vi "SigGenPwrMtr2.vi"() -> ()   [LabVIEW 2009]
uses:
  Reversing_Switch.ctl
panel:
  out "Noise Source Verified":bool
  in  "Inside Noise Source":bool
  in  "mSec":i32=250
  out "Power returned (dBm)":dbl(graph)=-33.1308036
  in  "stop":bool
  in  "Tab Control":T1(tab)=enum."SWITCH SETTINGS"
  out "RF Power":bool
  in  "RF ON/OFF":bool
  in  "Power Level (dB)":dbl=-120.0
  in  "Frequency (GHz)":dbl=2.809
  in  "SigGen Settings":bool
  out "Freq (GHz)":dbl=2809000000.0 format="%#_10e"
  out "Power":dbl=-120.0
  out "SigGen Errors":errorcluster
  in  "Switch Settings":bool
  in  "IO Switch #2 Output":T2(ring)
  in  "Signal Out Input":T3(ring)
  in  "Signal Out Output":T4(ring)
  in  "Power Meter Switch Input":T5(ring)
  in  "Amplifier Switch":enum16{"Bypass Amp", "Include Amp"}(ring)
  out "Reversing Switch":bool=TRUE
  out "IO Switch #1":bool=TRUE
  out "IO Switch #2":bool=TRUE
  out "Signal Out":bool=TRUE
  out "Signal Source":bool=TRUE
  out "Power Meter":bool=TRUE
  out "Amp By Pass":bool=TRUE
  in  "Reversing Switch":T6
  in  "IO Swith #2 Input":T7(ring)
  in  "IO Switch #1 Input":T8(ring)
  in  "Power Meter Switch Output":T9(ring)
  in  "Signnal Source Input":T10(ring)
  in  "Signal Source Output":T11(ring)
  in  "IO Switch #1 Output":T12(ring)
  out "Switch Errors":errorcluster
  in  "Attenuator Settings":bool
  in  "121 dB Attenuator":i32=121 min=0 max=121 step=1
  out "Active 121 dB Attenuators":bool[](array[boolean])=[FALSE, TRUE, TRUE, TRUE, TRUE, TRUE, TRUE, TRUE, TRUE]
  in  "70 dB Attenuator":i32=70 min=0 max=70 step=10
  out "Active 70 dB Attenuators":bool[](array[boolean])=[FALSE, TRUE, TRUE, TRUE]
  out "Attenuator Errors":errorcluster
  # "1 dB"
  # "2 dB"
  # "4 dB"
  # "4 dB"
  # "10 dB"
  # "20 dB"
  # "40 dB"
  # "40 dB"
  # "10 dB"
  # "20 dB"
  # "40 dB"
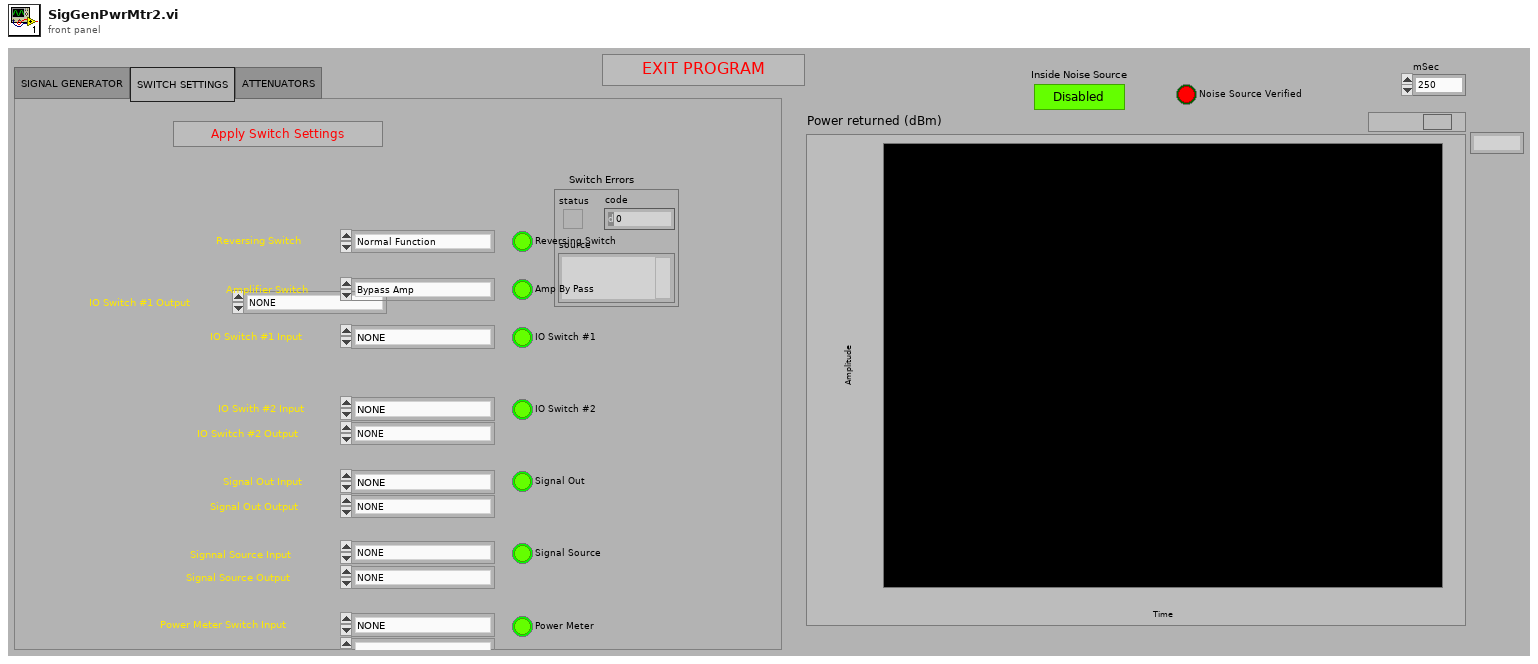
[diagram p1: front panel]
types:
  T1 = enum32{"SIGNAL GENERATOR", "SWITCH SETTINGS", "ATTENUATORS"}
  T2 = enum16{"NONE", "AVR (J3)", "Signal Out Switch (S3)", "Power Meter Switch (S5)", "Reversing Switch", "2W Term (TM1)"}
  T3 = enum16{"NONE", "Amp Bypass Switch (S6)", "IO Switch #1 (S1)", "IO Switch #2 (S2)", "2W Term (TM3)"}
  T4 = enum16{"NONE", "2 Watt Term (TM3)", "Splitter", "Power Meter Switch (S5)"}
  T5 = enum16{"NONE", "IO Switch #1 (S1)", "Signal Source Switch (S4)", "Signal Out Switch (S3)", "IO Switch #2 (S2)", "TXH-TXV Switch (J8)"}
  T6 = typedef "Reversing_Switch.ctl" = enum16{"Normal Function", "Reversing Function"}
  T7 = enum16{"NONE", "AVR (J3)", "Splitter", "Signal Out Switch (S3)", " 2W Term (TM1)", "Reversing Switch", "Power Meter Switch"}
  T8 = enum16{"NONE", "AHR (J2)", "Splitter", "Signal Out Switch (S3)", "Reversing Switch", "Power Meter Switch"}
  T9 = enum16{"NONE", "Power Meter (J6)", "IO Switch # 1", "IO Switch # 2"}
  T10 = enum16{"NONE", "Delay Device", "Signal Generator (J7)", "Inside Noise Box NF (J5)", "2W Term (TM3)"}
  T11 = enum16{"NONE", "Amp Bypass Switch", "Test Pulse Generator", "Power Meter Switch (S5)"}
  T12 = enum16{"NONE", "AHR (J2)", "Delay Device (S4)", "Power Meter Switch (S5)", "Reversing Switch"}
  T13 = enum16{"N1911A", "Siggen", "34980a", "E4418B", "Rvp8"}
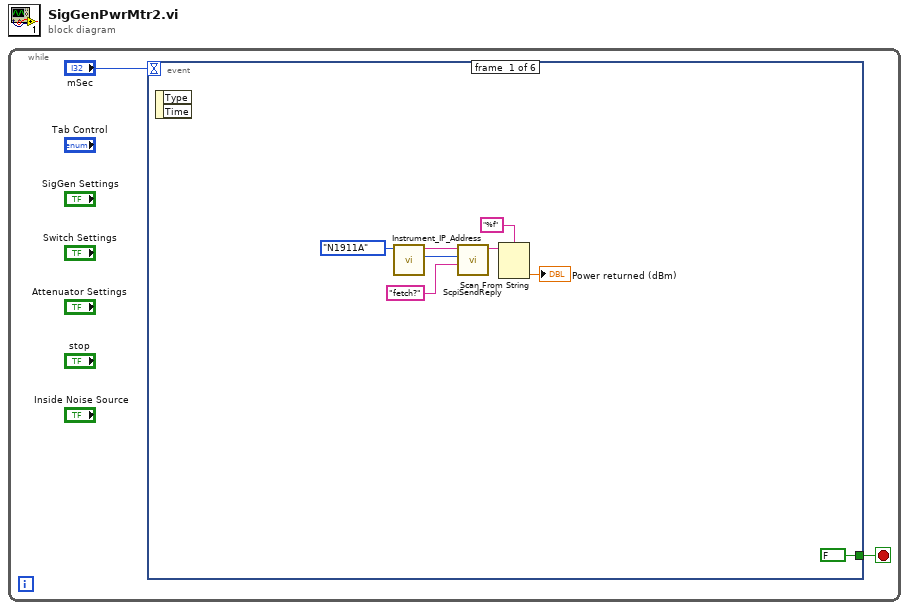
[diagram p0: block diagram]
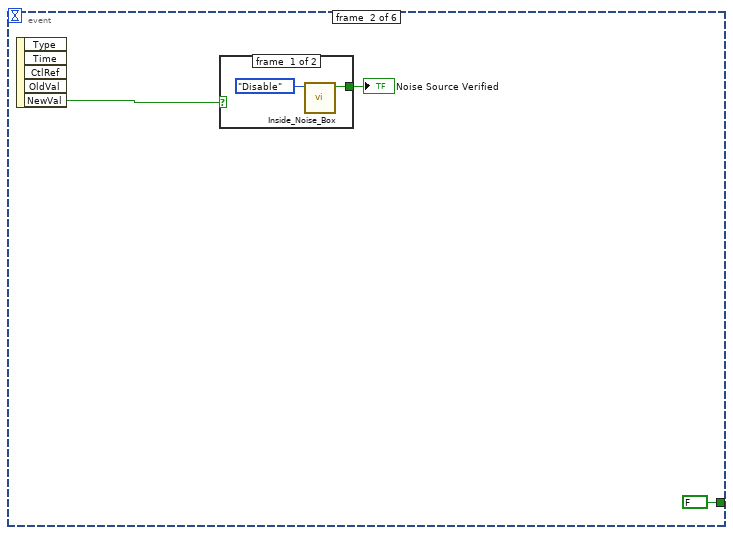
[diagram p2: hidden frame]
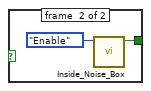
[diagram p3: hidden frame]
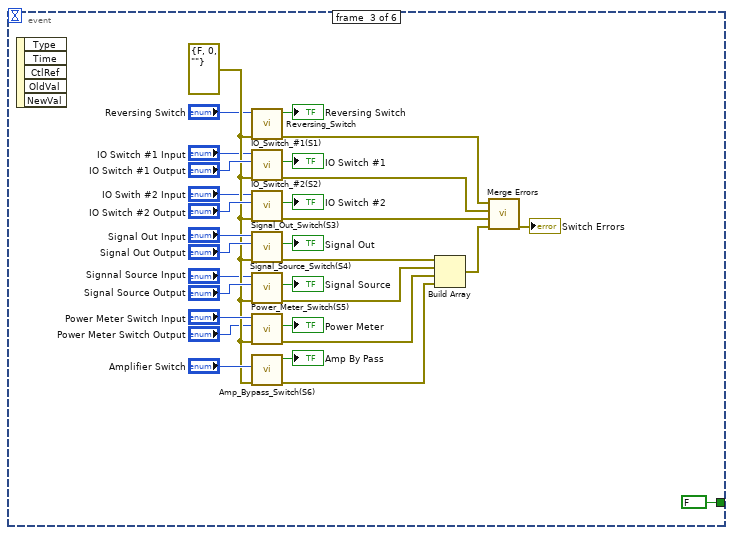
[diagram p4: hidden frame]
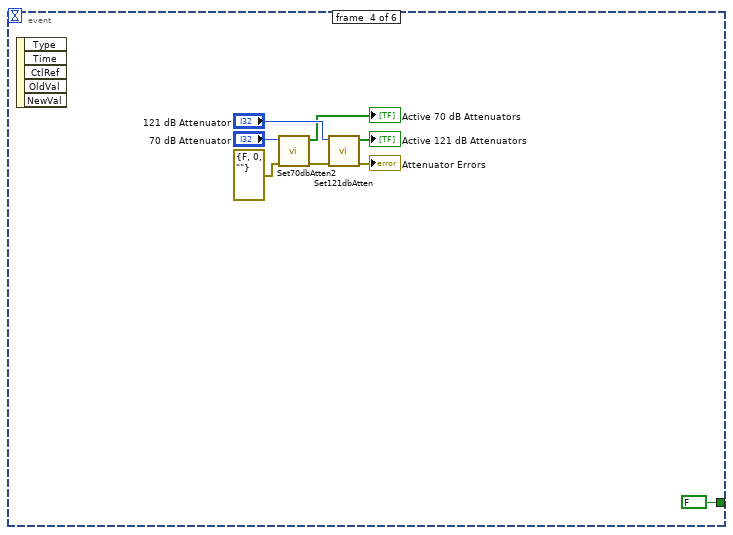
[diagram p5: hidden frame]
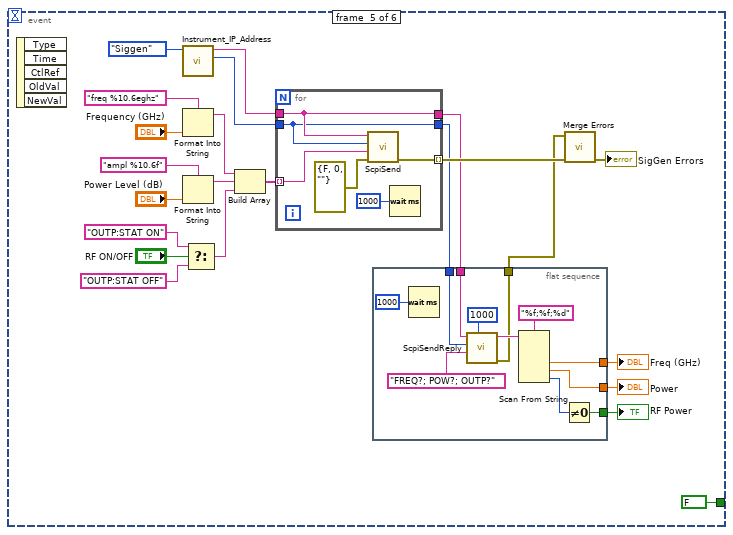
[diagram p6: hidden frame]
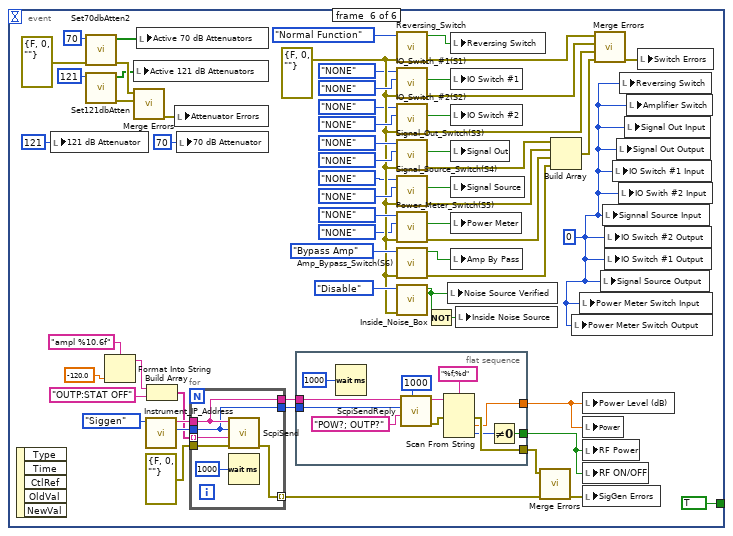
[diagram p7: hidden frame]
diagram:
  n1 = while {
    stop <- w2 stop-if-true
    n2 = event shown="[5] \"stop\": Value Change" {
      selector: _ -> [_ _ _ _ _ _]
      dyn-events: _ -> [_ _ _ _ _ _]
      timeout: "mSec" -> [_ _ _ _ _ _]
      tunnel: [FALSE FALSE FALSE FALSE FALSE TRUE] -> w2
      event #0 {
        n3 = event-data() -> ()  [unwired: 1 in, 2 out]
        n4 = call "Instrument_IP_Address.vi"("Instrument"=T13."N1911A") -> ("Port"=w10:u16, "IP Address"=w9:string)  [unwired: 9 in]
        n5 = call "ScpiSendReply.vi"("Command"="fetch?" ("format string"), "TCP port"=w10, "IP Address"=w9) -> ("Reply"=w5:string)  [unwired: 6 in, 1 out]
        n6 = Scan From String(format string="%f", input string=w5) -> (output 1=→"Power returned (dBm)":dbl)  [unwired: 3 in, 3 out]
      }
      event #1 {
        n7 = event-data() -> ("NewVal"=w13:bool)  [unwired: 1 in, 4 out]
        n8 = case shown="False" w13 {
          tunnel: [w14 w16] -> w12
          frame #0 {
            n9 = call "Inside_Noise_Box.vi"("Noise Switch Function"=enum16{"Disable", "Enable"}."Disable") -> ("Verfied"=w14:bool)  [unwired: 9 in, 1 out]
          }
          frame #1 {
            n10 = call "Inside_Noise_Box.vi"("Noise Switch Function"=enum16{"Disable", "Enable"}."Enable") -> ("Verfied"=w16:bool)  [unwired: 9 in, 1 out]
          }
        }
        "Noise Source Verified" <- w12
      }
      event #2 {
        w23 = errorcluster {"status"=FALSE, "code"=0, "source"=""} ("error in (no error)")
        n11 = event-data() -> ()  [unwired: 1 in, 5 out]
        n12 = call "Reversing_Switch.vi"("error in"=w23, "Reversing Switch Function"="Reversing Switch") -> ("error out"=w31:errorcluster, "Verfied"=→"Reversing Switch":bool)  [unwired: 8 in]
        n13 = call "IO_Switch_#1(S1).vi"("error in"=w23, "Output"="IO Switch #1 Output", "Input"="IO Switch #1 Input") -> ("error out"=w30:errorcluster, "Verfied"=→"IO Switch #1":bool)  [unwired: 6 in, 1 out]
        n14 = call "IO_Switch_#2(S2).vi"("error in"=w23, "Output"="IO Switch #2 Output", "Input"="IO Swith #2 Input") -> ("error out"=w29:errorcluster, "Verfied"=→"IO Switch #2":bool)  [unwired: 6 in, 1 out]
        n15 = call "Signal_Out_Switch(S3).vi"("error in"=w23, "Output"="Signal Out Output", "Input"="Signal Out Input") -> ("error out"=w28:errorcluster, "Verfied"=→"Signal Out":bool)  [unwired: 6 in, 1 out]
        n16 = call "Signal_Source_Switch(S4).vi"("error in"=w23, "Output"="Signal Source Output", "Input"="Signnal Source Input") -> ("error out"=w27:errorcluster, "Verfied"=→"Signal Source":bool)  [unwired: 6 in, 1 out]
        n17 = call "Power_Meter_Switch(S5).vi"("error in"=w23, "Output"="Power Meter Switch Output", "Input"="Power Meter Switch Input") -> ("error out"=w26:errorcluster, "Verfied"=→"Power Meter":bool)  [unwired: 6 in, 1 out]
        n18 = call "Amp_Bypass_Switch(S6).vi"("error in"=w23, "AMP Function"="Amplifier Switch") -> ("error out"=w25:errorcluster, "Verfied"=→"Amp By Pass":bool)  [unwired: 8 in]
        n19 = Build Array(w28, w27, w26, w25) -> (w33:errorcluster[])
        n20 = call <vilib>:"Merge Errors.vi"("error array in"=w33, "error in 3 (no error)"=w29, "error in 2 (no error)"=w30, "error in 1 (no error)"=w31) -> ("error out"=→"Switch Errors":errorcluster)  [unwired: 3 in]
      }
      event #3 {
        n21 = event-data() -> ()  [unwired: 1 in, 5 out]
        n22 = call "Set70dbAtten2.vi"("error in (no error)"=errorcluster {"status"=FALSE, "code"=0, "source"=""}, "Attenuation (dB)"="70 dB Attenuator") -> ("error out"=w49:errorcluster, "Active Attenuators"=→"Active 70 dB Attenuators":bool[])  [unwired: 7 in, 1 out]
        n23 = call "Set121dbAtten.vi"("error in (no error)"=w49, "Attenuation (dB)"="121 dB Attenuator") -> ("error out"=→"Attenuator Errors":errorcluster, "Active Attenuators"=→"Active 121 dB Attenuators":bool[])  [unwired: 7 in, 1 out]
      }
      event #4 {
        n24 = event-data() -> ()  [unwired: 1 in, 5 out]
        n25 = call "Instrument_IP_Address.vi"("Instrument"=T13."Siggen") -> ("Port"=w69:u16, "IP Address"=w68:string)  [unwired: 9 in]
        n26 = Format Into String(format string="freq %10.6eghz", "Frequency (GHz)") -> (resulting string=w73:string)  [unwired: 2 in, 1 out]
        n27 = Format Into String(format string="ampl %10.6f", "Power Level (dB)") -> (resulting string=w72:string)  [unwired: 2 in, 1 out]
        n28 = Select(t="OUTP:STAT ON" ("format string"), s="RF ON/OFF", f="OUTP:STAT OFF" ("format string")) -> (s? t:f=w71:string)
        n29 = Build Array(w73, w72, w71) -> (w70:string[])
        n30 = for {
          tunnel: w70 -> [w96] mode=indexing
          tunnel: w69 -> [w92]
          tunnel: w68 -> [w93]
          tunnel: [w93] -> w58
          tunnel: [w92] -> w57
          tunnel: [w91] -> w64 mode=indexing
          n31 = call "ScpiSend.vi"("error in (no error)"=errorcluster {"status"=FALSE, "code"=0, "source"=""}, "Command"=w96, "TCP port"=w92, "IP Address"=w93) -> ("error out"=w91:errorcluster)  [unwired: 7 in]
          n32 = Wait (ms)(milliseconds to wait=u32 1000) -> ()  [unwired: 1 out]
        }
        n33 = flat-sequence {
          tunnel: [w85] -> w62
          tunnel: [w84] -> w61
          tunnel: [w83] -> w60
          tunnel: [w82] -> w59
          tunnel: w58 -> [w80]
          tunnel: w57 -> [w79]
          frame #0 {
            n34 = Wait (ms)(milliseconds to wait=u32 1000) -> ()  [unwired: 1 out]
            n35 = call "ScpiSendReply.vi"("TCP Timeout mS"=1000, "Command"="FREQ?; POW?; OUTP?" ("format string"), "TCP port"=w79, "IP Address"=w80) -> ("Error out"=w82:errorcluster, "Reply"=w88:string)  [unwired: 5 in]
            n36 = Scan From String(format string="%f;%f;%d", input string=w88) -> (output 1=w83:dbl, output 2=w84:dbl, output 3=w90:i32)  [unwired: 5 in, 3 out]
            n37 = Not Equal To 0?(x=w90) -> (x != 0?=w85:bool)
          }
        }
        n38 = call <vilib>:"Merge Errors.vi"("error array in"=w64, "error in 1 (no error)"=w59) -> ("error out"=→"SigGen Errors":errorcluster)  [unwired: 5 in]
        "RF Power" <- w62
        "Freq (GHz)" <- w60
        "Power" <- w61
      }
      event #5 {
        w102 = u16 0
        w105 = errorcluster {"status"=FALSE, "code"=0, "source"=""} ("error in (no error)")
        n39 = event-data() -> ()  [unwired: 1 in, 5 out]
        n40 = local write "121 dB Attenuator"(121 ("121 dB Attenuator")) -> ()
        n41 = call "Set70dbAtten2.vi"("error in (no error)"=errorcluster {"status"=FALSE, "code"=0, "source"=""}, "Attenuation (dB)"=70) -> ("error out"=w155:errorcluster, "Active Attenuators"=w150:bool[])  [unwired: 7 in, 1 out]
        n42 = call "Set121dbAtten.vi"("Attenuation (dB)"=121) -> ("error out"=w154:errorcluster, "Active Attenuators"=w149:bool[])  [unwired: 8 in, 1 out]
        n43 = Format Into String(format string="ampl %10.6f", -120.0 ("input 1")) -> (resulting string=w116:string)  [unwired: 2 in, 1 out]
        n44 = local write "Active 121 dB Attenuators"(w149) -> ()
        n45 = call <vilib>:"Merge Errors.vi"("error in 2 (no error)"=w154, "error in 1 (no error)"=w155) -> ("error out"=w148:errorcluster)  [unwired: 5 in]
        n46 = local write "Active 70 dB Attenuators"(w150) -> ()
        n47 = call "Instrument_IP_Address.vi"("Instrument"=T13."Siggen") -> ("Port"=w121:u16, "IP Address"=w122:string)  [unwired: 9 in]
        n48 = Build Array(w116, "OUTP:STAT OFF" ("format string")) -> (w114:string[])
        n49 = local write "Attenuator Errors"(w148) -> ()
        n50 = local write "70 dB Attenuator"(70 ("70 dB Attenuator")) -> ()
        n51 = for {
          tunnel: errorcluster {"status"=FALSE, "code"=0, "source"=""} ("error in (no error)") -> [w162]
          tunnel: w122 -> [w159]
          tunnel: w121 -> [w158]
          tunnel: [w161] -> w110 mode=indexing
          tunnel: w114 -> [w160] mode=indexing
          tunnel: [w159] -> w113
          tunnel: [w158] -> w112
          n52 = call "ScpiSend.vi"("error in (no error)"=w162, "Command"=w160, "TCP port"=w158, "IP Address"=w159) -> ("error out"=w161:errorcluster)  [unwired: 7 in]
          n53 = Wait (ms)(milliseconds to wait=u32 1000) -> ()  [unwired: 1 out]
        }
        n54 = flat-sequence {
          tunnel: [w171] -> w107
          tunnel: w113 -> [w169]
          tunnel: [w167] -> w109
          tunnel: w112 -> [w166]
          tunnel: [w163] -> w108
          frame #0 {
            n55 = Wait (ms)(milliseconds to wait=u32 1000) -> ()  [unwired: 1 out]
            n56 = call "ScpiSendReply.vi"("TCP Timeout mS"=1000, "Command"="POW?; OUTP?" ("format string"), "TCP port"=w166, "IP Address"=w169) -> ("Error out"=w168:errorcluster, "Reply"=w174:string)  [unwired: 5 in]
            n57 = Scan From String(format string="%f;%d", input string=w174, error in=w168) -> (error out=w167:errorcluster, output 1=w163:dbl, output 2=w164:i32)  [unwired: 3 in, 2 out]
            n58 = Not Equal To 0?(x=w164) -> (x != 0?=w171:bool)
          }
        }
        n59 = call "Reversing_Switch.vi"("error in"=w105, "Reversing Switch Function"=Reversing_Switch."Normal Function") -> ("error out"=w142:errorcluster, "Verfied"=w132:bool)  [unwired: 8 in]
        n60 = call "IO_Switch_#1(S1).vi"("error in"=w105, "Output"=T12."NONE", "Input"=T8."NONE") -> ("error out"=w141:errorcluster, "Verfied"=w131:bool)  [unwired: 6 in, 1 out]
        n61 = call "IO_Switch_#2(S2).vi"("error in"=w105, "Output"=T2."NONE", "Input"=T7."NONE") -> ("error out"=w140:errorcluster, "Verfied"=w130:bool)  [unwired: 6 in, 1 out]
        n62 = call "Signal_Out_Switch(S3).vi"("error in"=w105, "Output"=T4."NONE", "Input"=T3."NONE") -> ("error out"=w144:errorcluster, "Verfied"=w129:bool)  [unwired: 6 in, 1 out]
        n63 = call "Signal_Source_Switch(S4).vi"("error in"=w105, "Output"=T11."NONE", "Input"=T10."NONE") -> ("error out"=w145:errorcluster, "Verfied"=w128:bool)  [unwired: 6 in, 1 out]
        n64 = call "Power_Meter_Switch(S5).vi"("error in"=w105, "Output"=T9."NONE", "Input"=T5."NONE") -> ("error out"=w146:errorcluster, "Verfied"=w127:bool)  [unwired: 6 in, 1 out]
        n65 = call "Amp_Bypass_Switch(S6).vi"("error in"=w105, "AMP Function"=enum16{"Bypass Amp", "Include Amp"}."Bypass Amp") -> ("error out"=w147:errorcluster, "Verfied"=w126:bool)  [unwired: 8 in]
        n66 = call "Inside_Noise_Box.vi"("error in"=w105, "Noise Switch Function"=enum16{"Disable", "Enable"}."Disable") -> ("Verfied"=w103:bool)  [unwired: 8 in, 1 out]
        n67 = Not(x=w103) -> (.not. x?=w104:bool)
        n68 = local write "Noise Source Verified"(w103) -> ()
        n69 = local write "Reversing Switch"(w132) -> ()
        n70 = local write "IO Switch #1"(w131) -> ()
        n71 = local write "IO Switch #2"(w130) -> ()
        n72 = local write "Signal Out"(w129) -> ()
        n73 = local write "Signal Source"(w128) -> ()
        n74 = local write "Power Meter"(w127) -> ()
        n75 = local write "Amp By Pass"(w126) -> ()
        n76 = local write "Inside Noise Source"(w104) -> ()
        n77 = call <vilib>:"Merge Errors.vi"("error array in"=w110, "error in 1 (no error)"=w109) -> ("error out"=w111:errorcluster)  [unwired: 5 in]
        n78 = Build Array(w144, w145, w146, w147) -> (w143:errorcluster[])
        n79 = local write "Power Meter Switch Output"(w102) -> ()
        n80 = local write "Power Meter Switch Input"(w102) -> ()
        n81 = local write "Power Level (dB)"(w108) -> ()
        n82 = local write "Power"(w108) -> ()
        n83 = local write "RF Power"(w107) -> ()
        n84 = local write "RF ON/OFF"(w107) -> ()
        n85 = local write "SigGen Errors"(w111) -> ()
        n86 = call <vilib>:"Merge Errors.vi"("error array in"=w143, "error in 3 (no error)"=w140, "error in 2 (no error)"=w141, "error in 1 (no error)"=w142) -> ("error out"=w125:errorcluster)  [unwired: 3 in]
        n87 = local write "Signal Source Output"(w102) -> ()
        n88 = local write "Signnal Source Input"(w102) -> ()
        n89 = local write "IO Switch #2 Output"(w102) -> ()
        n90 = local write "IO Switch #1 Output"(w102) -> ()
        n91 = local write "IO Switch #1 Input"(w102) -> ()
        n92 = local write "Signal Out Output"(w102) -> ()
        n93 = local write "IO Swith #2 Input"(w102) -> ()
        n94 = local write "Reversing Switch"(w102) -> ()
        n95 = local write "Signal Out Input"(w102) -> ()
        n96 = local write "Amplifier Switch"(w102) -> ()
        n97 = local write "Switch Errors"(w125) -> ()
      }
    }
  }
